vi "okCFrontPanel Dispose Device.vi"(8 "Error In":errorcluster, 11 "okCFrontPanel Refnum":refnum<k24>) -> (0 "Error Out":errorcluster)   [LabVIEW 2021, in "okFrontPanelC#Wrapper.lvlib"]
uses:
  okFrontPanelC#Wrapper.lvlib
  D:/UCLA Thinkpad Google Drive/LabVIEW 2021 SP1/builds/SwissSPAD Live Distribution/Opal Kelly/C# Wrapper/v5.0.2/libFrontPanel-csharp.dll
  v5.0.2/libFrontPanel-csharp.dll
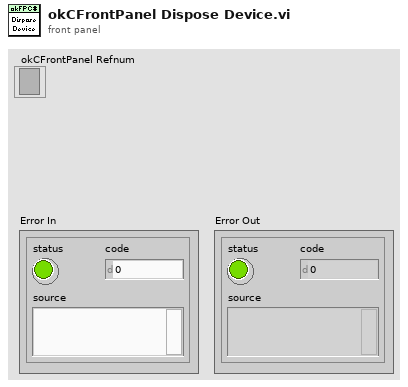
[diagram p1: front panel]
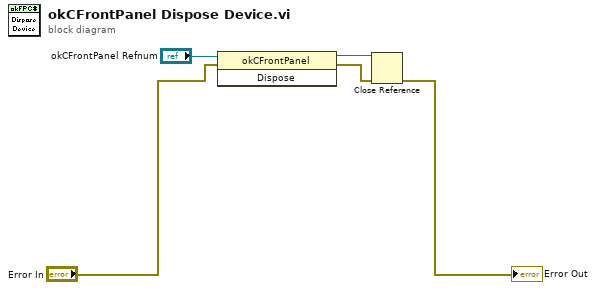
[diagram p0: block diagram]
diagram:
  n1 = invoke class="okCFrontPanel" method="Dispose"(reference="okCFrontPanel Refnum", error in="Error In") -> (reference out=w1:refnum<k24>, error out=w2:errorcluster)  [unwired: 1 in, 1 out]
  n2 = Close Reference(reference=w1, error in (no error)=w2) -> (error out=→"Error Out":errorcluster)
